vi "System@DynamicPanelBG__Parameter.vi"(1 "ParamterIn":string) -> (0 "ParamterOut":string)   [LabVIEW 2020]
uses:
  MainFrame/Global.vi
panel:
  out "Image":T1(plugin-control)
  in  "Picture":string(combo)
  in  "Confirm":bool
  # "System@DynamicPanelBG $Picture"
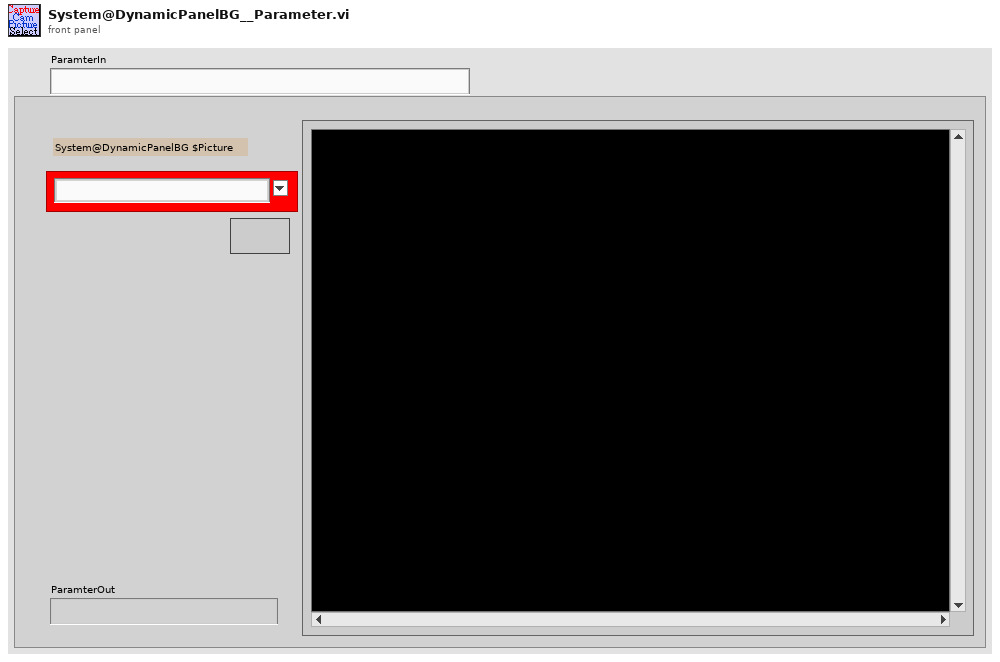
[diagram p1: front panel]
types:
  T1 = typedef "IMAQ Image.ctl" = refnum<image>
  T2 = typedef "Image Type" = u32
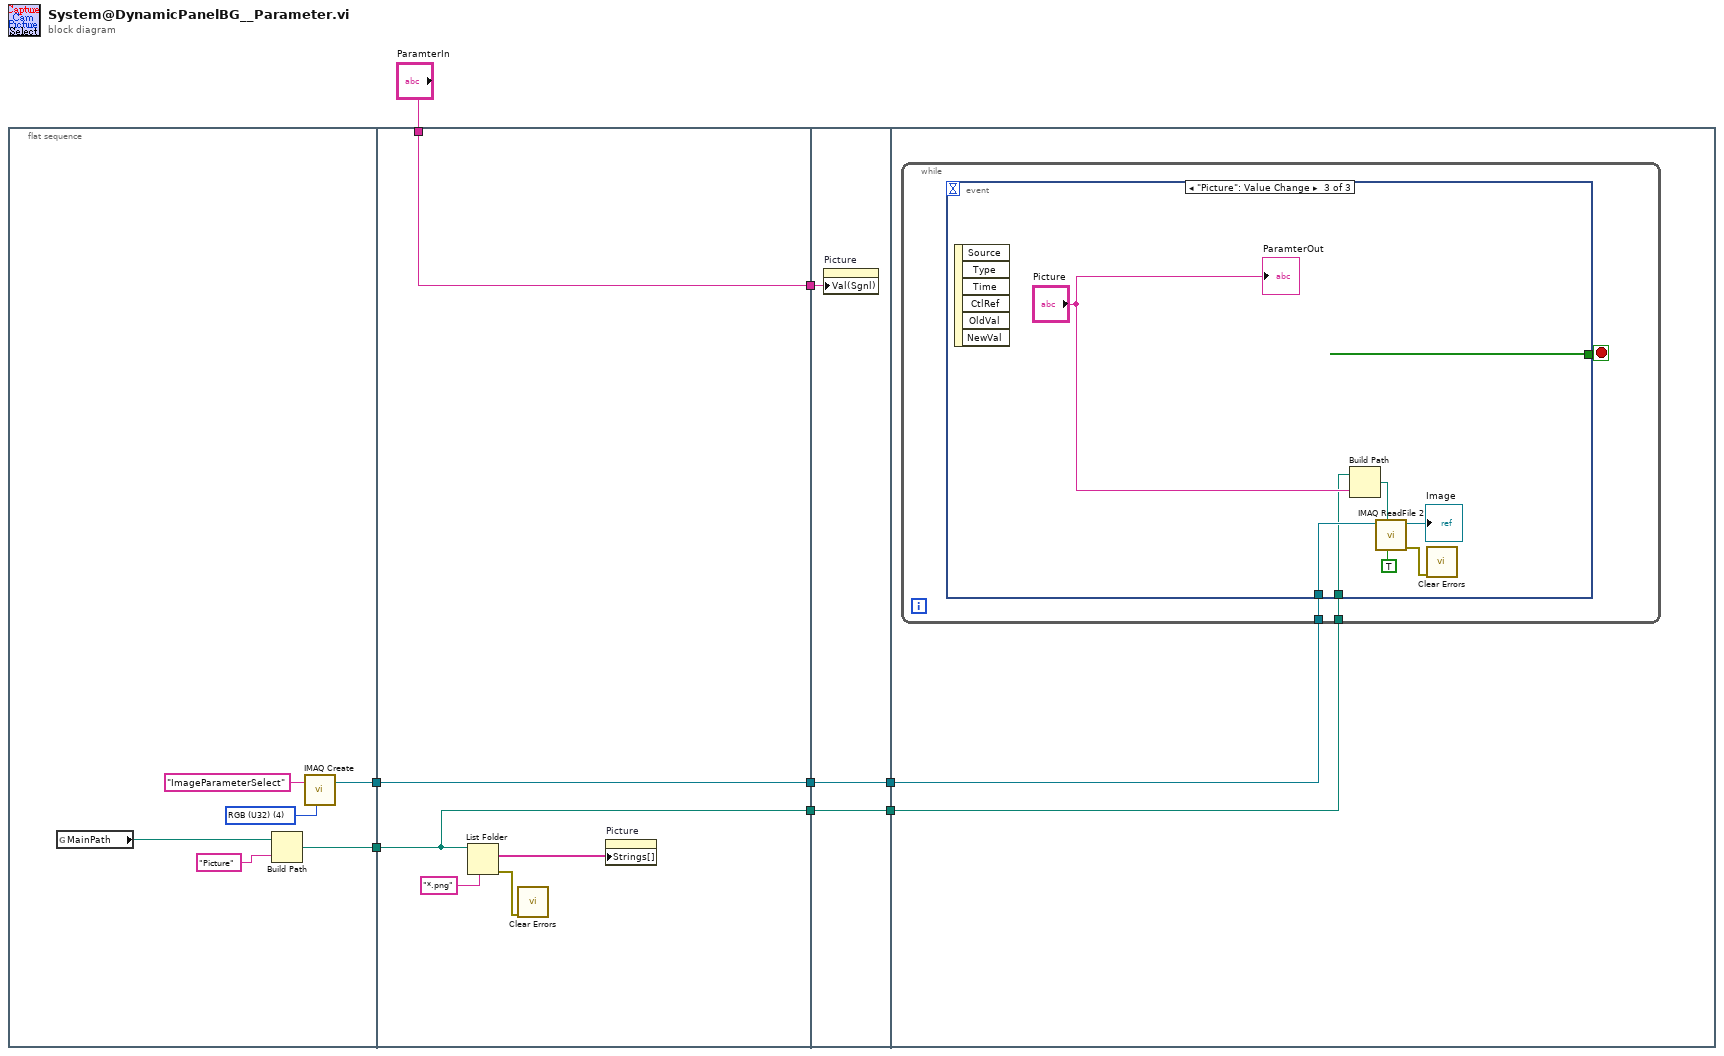
[diagram p0: block diagram]
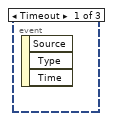
[diagram p2: hidden frame]
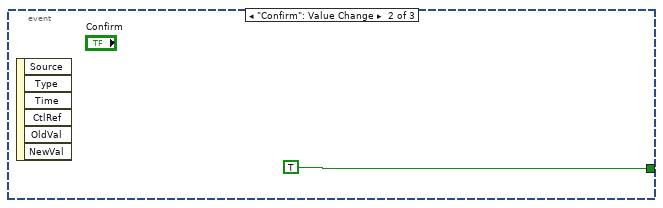
[diagram p3: hidden frame]
diagram:
  n1 = flat-sequence {
    tunnel: [w13] -> w7
    tunnel: [w11] -> w4
    tunnel: "ParamterIn" -> [w16]
    tunnel: w7 -> [w20]
    tunnel: [w20] -> w6
    tunnel: w4 -> [w17]
    tunnel: [w16] -> w3
    tunnel: [w17] -> w1
    tunnel: w6 -> [w23]
    tunnel: [w23] -> w5
    tunnel: w3 -> [w22]
    tunnel: [w21] -> w2
    tunnel: w1 -> [w21]
    tunnel: w5 -> [w25]
    tunnel: w2 -> [w24]
    frame #0 {
      w9 = T2 4 items=["Grayscale (U8)", "Grayscale (I16)", "Grayscale (SGL)", "Complex (CSG)", "RGB (U32)", "HSL (U32)", "RGB (U64)", "Grayscale (U16)"] ("Image Type")
      n2 = global read "Global.vi" "MainPath"() -> (w10:path)
      n3 = Build Path(base path=w10, name or relative path="Picture") -> (appended path=w11:path)
      n4 = call "IMAQ Create"("Image Name"="ImageParameterSelect", "Image Type"=w9) -> ("New Image"=w13:T1)  [unwired: 3 in, 1 out]
    }
    frame #1 {
      n5 = List Folder(path=w17, pattern="*.png") -> (filenames=w15:string[], error out=w19:errorcluster)  [unwired: 2 in, 2 out]
      n6 = call <vilib>:"Clear Errors.vi"("error in (no error)"=w19) -> ()  [unwired: 5 in, 2 out]
      n7 = property on="Picture" class="CmbBox"("Strings[]"=w15) -> ()  [unwired: 2 in, 2 out]
    }
    frame #2 {
      n8 = property on="Picture" class="CmbBox"("Val(Sgnl)"=w22) -> ()  [unwired: 2 in, 2 out]
    }
    frame #3 {
      n9 = while {
        tunnel: w25 -> [w27]
        tunnel: w24 -> [w26]
        stop <- w28 stop-if-true
        n10 = event shown="[2] \"Picture\": Value Change" {
          selector: _ -> [_ _ _]
          dyn-events: _ -> [_ _ _]
          timeout: _ -> [_ _ _]
          tunnel: [_ TRUE _] -> w28
          tunnel: w27 -> [_ _ w36]
          tunnel: w26 -> [_ _ w30]
          event Timeout {
            n11 = event-data() -> ()  [unwired: 1 in, 3 out]
          }
          event "Confirm": Value Change {
            n12 = event-data() -> ()  [unwired: 1 in, 6 out]
          }
          event "Picture": Value Change {
            n13 = event-data() -> ()  [unwired: 1 in, 6 out]
            n14 = Build Path(base path=w30, name or relative path="Picture") -> (appended path=w35:path)
            n15 = call "IMAQ ReadFile 2"("Use File Path Image Type"=TRUE, "File Path"=w35, "Image"=w36) -> ("error out"=w34:errorcluster, "Image Out"=→"Image":T1)  [unwired: 4 in, 3 out]
            n16 = call <vilib>:"Clear Errors.vi"("error in (no error)"=w34) -> ()  [unwired: 5 in, 2 out]
            "ParamterOut" <- "Picture"
          }
        }
      }
    }
  }
